vi "ex6.vi"() -> ()   [LabVIEW 2022 SP3]
panel:
  out "offset past match":i32
  in  "String":string
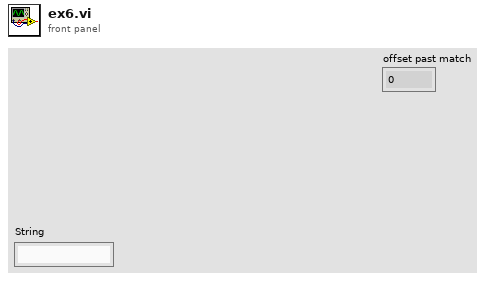
[diagram p1: front panel]
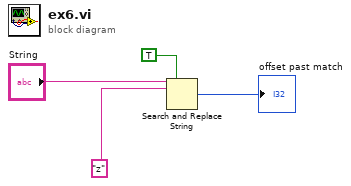
[diagram p0: block diagram]
diagram:
  n1 = Search and Replace String(replace all?=TRUE ("replace all? (F)"), input string="String", search string="z" ("regular expression")) -> (number of replacements=→"offset past match":i32)  [unwired: 5 in, 3 out]
